vi "Colores_Escada.vi"() -> ()   [LabVIEW 2016]
panel:
  out "Array":u32[](array[colorbox])
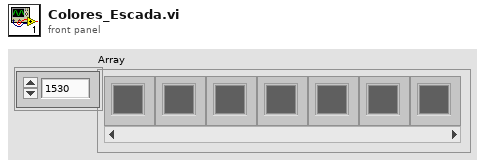
[diagram p1: front panel]
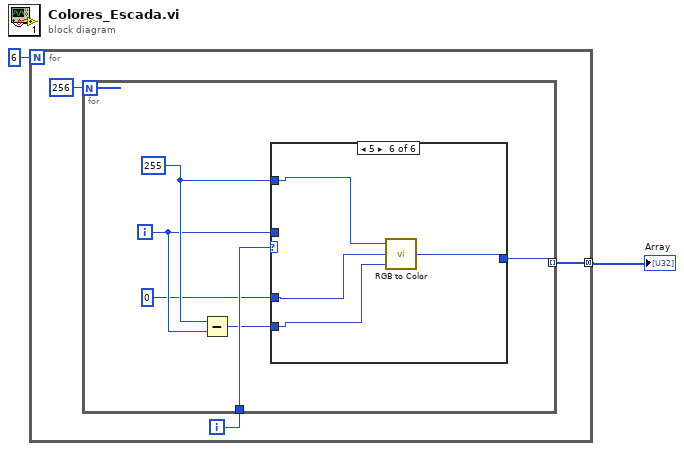
[diagram p0: block diagram]
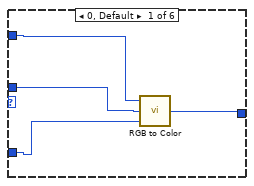
[diagram p2: hidden frame]
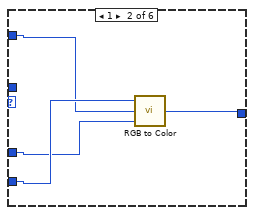
[diagram p3: hidden frame]
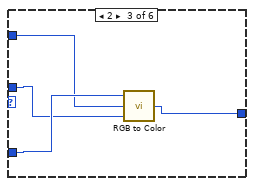
[diagram p4: hidden frame]
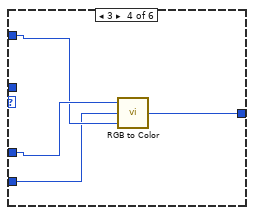
[diagram p5: hidden frame]
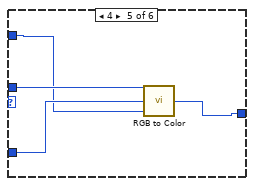
[diagram p6: hidden frame]
diagram:
  n1 = for {
    N: 6 -> [_]
    tunnel: [w3] -> w1 mode=concatenating
    i -> [w4]
    n2 = for {
      N: 256 -> [_]
      tunnel: w4 -> [w11]
      tunnel: [w6] -> w3 mode=indexing
      i -> [w9]
      w10 = i16 255 ("x")
      n3 = Subtract(x=w10, y=w9) -> (x-y=w7:i32)
      n4 = case shown="5" w11 {
        tunnel: w10 -> [w15 w18 w22 w26 w29 w35]
        tunnel: w9 -> [w14 _ w21 _ w31 _]
        tunnel: i16 0 ("x") -> [w13 w17 w23 w27 w30 w34]
        tunnel: w7 -> [_ w19 _ w25 _ w33]
        tunnel: [w12 w16 w20 w24 w28 w32] -> w6
        frame 0, Default {
          n5 = call <vilib>:"RGB to Color.vi"("B"=w13, "G"=w14, "R"=w15) -> ("Color"=w12:u32)
        }
        frame 1 {
          n6 = call <vilib>:"RGB to Color.vi"("B"=w17, "G"=w18, "R"=w19) -> ("Color"=w16:u32)
        }
        frame 2 {
          n7 = call <vilib>:"RGB to Color.vi"("B"=w21, "G"=w22, "R"=w23) -> ("Color"=w20:u32)
        }
        frame 3 {
          n8 = call <vilib>:"RGB to Color.vi"("B"=w26, "G"=w25, "R"=w27) -> ("Color"=w24:u32)
        }
        frame 4 {
          n9 = call <vilib>:"RGB to Color.vi"("B"=w29, "G"=w30, "R"=w31) -> ("Color"=w28:u32)
        }
        frame 5 {
          n10 = call <vilib>:"RGB to Color.vi"("B"=w33, "G"=w34, "R"=w35) -> ("Color"=w32:u32)
        }
      }
    }
  }
  "Array" <- w1
